vi "Test List Tests from lvlib Includes top Level Suite.vi"(8 "error in (no error)":errorcluster, 11 "Test Case In":refnum<class "LUnit Test Suite Tests.lvclass">) -> (0 "error out":errorcluster, 3 "Test Case Out":refnum<class "LUnit Test Suite Tests.lvclass">)   [LabVIEW 2020, in "LUnit Test Suite Tests.lvclass"]
uses:
  LUnit Test Suite Tests.lvclass
  C:/Program Files (x86)/National Instruments/LabVIEW 2020/vi.lib/Astemes/LUnit/Test Case.lvclass
  source/Core/Result/Result.ctl
  source/Core/Result/Status.ctl
  source/Core/Result/Type.ctl
  <vilib>/Astemes/LUnit/Test Case.lvclass/Test Case.ctl
  f811901c-9033-46b2-854c-adcdfd14f7b8.vi
  <vilib>/Astemes/LUnit/Palette/Pass If.vi
  <vilib>/Astemes/LUnit/Core/LUnit Test Case/Private/Append Fail Result.vi
  <vilib>/Astemes/LUnit/Core/LUnit Test Case/Private/Append Pass Result.vi
  <vilib>/Astemes/LUnit/Core/LUnit Test Case/Private/Run In UI.vi
  <vilib>/Utility/error.llb/Clear Errors.vi
  source/LUnit Test Suite.lvclass
  C:/git/astemes-lunit/source/Runnable.lvclass
  source/Framework/Test Suite Factory/Test Suite Factory.lvclass
  source/Runnable.lvclass
  source/Core/Result/Result.lvlib
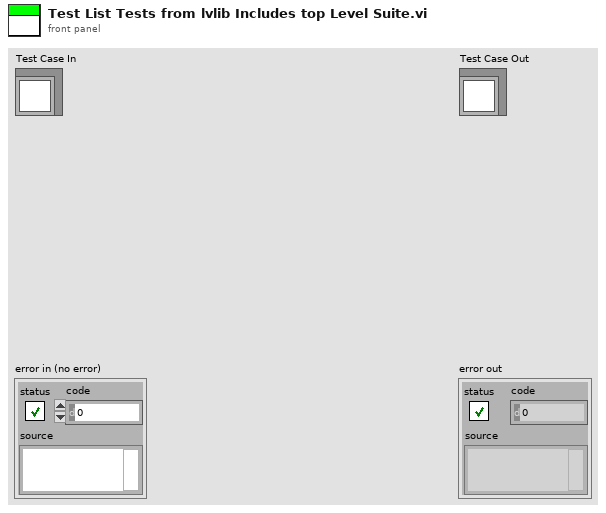
[diagram p1: front panel]
types:
  T1 = typedef "Result.lvlib/Result.ctl" = cluster{"Name":string, "Description":string, "Status":T2, "Result Type":T3, "Execution Time":dbl, "Data":cluster{"Expected":variant, "Actual":variant, "Delta":variant}}
  T2 = typedef "Result.lvlib/Status.ctl" = enum16{"", "Passed", "Failed", "Error", "Skipped", "Setup Error", "Broken", "Teardown Error"}
  T3 = typedef "Result.lvlib/Type.ctl" = enum16{"Test Case", "Test Suite", "Test Run", "Pass", "Fail", "Skip", "Pass if", "Fail if", "Pass if Error", "Fail if Error", "Pass if Equal", "Fail if Equal"}
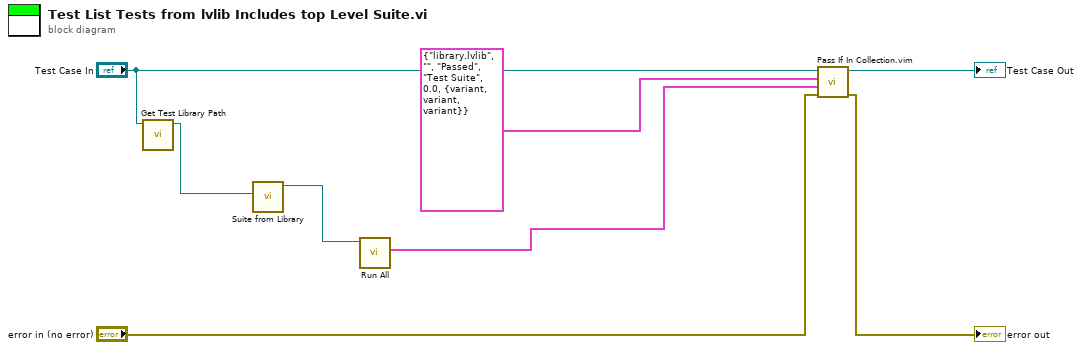
[diagram p0: block diagram]
diagram:
  n1 = call "Get Test Library Path.vi"("LUnit Test Suite Tests in"="Test Case In") -> ("lvlib path"=w4:path)  [unwired: 9 in, 1 out]
  n2 = call "Suite from Library.vi"("Library Path"=w4) -> ("LUnit Test Suite Out"=w3:refnum<class "LUnit Test Suite.lvclass">)  [unwired: 9 in, 1 out]
  n3 = call "Run All.vi"("Runnable In"=w3) -> ("Results"=w2:T1[])  [unwired: 9 in, 1 out]
  n4 = call "Pass If In Collection.vim"("error in (no error)"="error in (no error)", "Collection"=w2, "Expected Element"=T1 {"Name"="library.lvlib", "Description"="", "Status"=enum."Passed", "Result Type"=enum."Test Suite", "Execution Time"=0.0, "Data"={"Expected"=variant, "Actual"=variant, "Delta"=variant}} ("Result"), "LUnit Test Case In"="Test Case In") -> ("error out"=→"error out":errorcluster, "LUnit Test Case Out"=→"Test Case Out":refnum<class "LUnit Test Suite Tests.lvclass">)  [unwired: 6 in]
